vi "Create VS Engine.vi"(8 "error in":errorcluster, 11 "Custom Device Item Ref":T1=18446744073709551615 format="%.0x") -> (0 "error out":errorcluster, 3 "VS Engine out":refnum<class "VS Engine.lvclass">)   [LabVIEW 2024, in "VS Engine Abstraction.lvlib" / "VS Engine.lvclass"]
uses:
  VS Engine.lvclass
  <vilib>/NI VeriStand/Custom Device API/Custom Device Item Ref.ctl
  VS Engine.lvclass/VS Engine.ctl
  <vilib>/NI VeriStand/Custom Device API/Custom Device API.lvlib
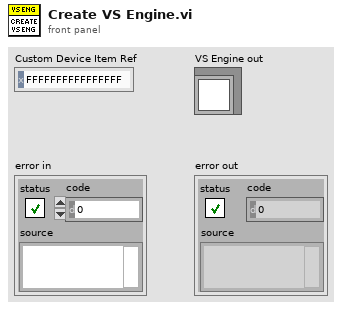
[diagram p1: front panel]
types:
  T1 = typedef "Custom Device API.lvlib/Custom Device Item Ref.ctl" = u64
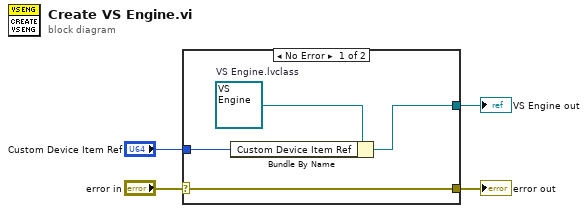
[diagram p0: block diagram]
diagram:
  n1 = case shown="No Error" "error in" {
    selector: "error in" -> [w8 w9]
    tunnel: [w8 w9] -> w3
    tunnel: "Custom Device Item Ref" -> [w7 _]
    tunnel: [w5 _] -> w1
    frame No Error {
      w6 = refnum<class "VS Engine.lvclass"> refnum  # VS Engine.lvclass
      n2 = Bundle By Name(cluster=w6, "Custom Device Item Ref"=w7) -> (w5:refnum<class "VS Engine.lvclass">)
    }
    frame Error {
    }
  }
  "error out" <- w3
  "VS Engine out" <- w1
